vi "Dashboard Main.vi"() -> ()   [LabVIEW 2018]
uses:
  <vilib>/event_ctls.llb/eventvkey.ctl
  <vilib>/Rock Robotics/WPI/Dashboard/WPI_DashboardLogging Global.vi
  <vilib>/Utility/miscctls.llb/LVRowAndColumnTypeDef.ctl
  <vilib>/Rock Robotics/Network Tables/NT Read Boolean.vi
  7eadb382-1a2a-4737-94d3-f53f3babfc2e.vi
  <vilib>/Rock Robotics/Network Tables/NT Read Numeric Array.vi
  <vilib>/Utility/file.llb/Read Delimited Spreadsheet (string).vi
panel:
  in  "DB Camera Config 2":bool
  out "Camera Perf":string
  in  "Camera Settings":T1={"Frame Rate"=30, "Compression"=30, "Size"=1} {"Frame Rate" scale=1.0..30.0; "Compression" scale=100.0..-1.0; "Size" items=["640x480", "320x240", "160x120"]}
  in  "TCP":refnum<k5>
  out "Robot IP":string
  out "Image Message":string="Timeout in Camera Communications"
  in  "Dashboard Tab":T2(tab)
  in  "DB Camera Config":bool
  out "NT Connection":bool
  out "MotorChart R":cluster{"Numeric":dbl, "Numeric":dbl}(graph)
  out "MotorChart L":cluster{"Numeric":dbl, "Numeric":dbl}(graph)
  out "MotorSliders R":cluster{"MotorSlide1":dbl, "MotorSlide2":dbl} {"MotorSlide2" scale=-1.0..1.0 scale format="%#_2e"; "MotorSlide1" scale=-1.0..1.0 scale format="%#_2e"}
  out "MotorSliders L":cluster{"MotorSlide1":dbl, "MotorSlide2":dbl} {"MotorSlide2" scale=-1.0..1.0 scale format="%#_2e"; "MotorSlide1" scale=-1.0..1.0 scale format="%#_2e"}
  out "JS1 Z":dbl(slide) scale=-1.0..1.0 scale format="%#_2e"
  out "JS1 Graph":cluster{"X":dbl, "Y":dbl}[](graph)
  out "JS1 Buttons":T3
  out "JS2 Z":dbl(slide) scale=-1.0..1.0 scale format="%#_2e"
  out "JS2 Graph":cluster{"X":dbl, "Y":dbl}[](graph)
  out "JS2 Buttons":T3
  out "Mode":T4(ring)=enum."Auto Disabled"
  out "Right Camera Perf":cluster{"Bandwidth (Mbps)":dbl, "FPS":dbl}
  in  "Camera Name Right":string(combo)="No Camera Selection"
  in  "Camera Settings Right":T1={"Frame Rate"=30, "Compression"=30, "Size"=1} {"Frame Rate" scale=1.0..30.0; "Compression" scale=100.0..-1.0; "Size" items=["640x480", "320x240", "160x120"]}
  in  "Rec Mode":enum32{"Stop", "Record", "Playback"}(radio)
  in  "RIGHT TRAIN file path for Motion Profile Tester":path=path "C:/Users/Robotics/Desktop/2019 Deep Space/Motion Profile Examples and Resources/Phoenix-Examples-LabVIEW-master/MotionProfile (Edited by Drake)/mp.csv"
  out "RIGHT Trajectory Pts from .csv File":dbl[][](array[numeric])
  in  "Read New Profile for Tester":bool
  in  "LEFT TRAIN file path for Motion Profile Tester":path=path "C:/Users/Robotics/Desktop/2019 Deep Space/Motion Profile Examples and Resources/Phoenix-Examples-LabVIEW-master/MotionProfile (Edited by Drake)/mp.csv"
  out "LEFT Trajectory Pts from .csv File":dbl[][](array[numeric])
  out "Camera Image Right":T5(plugin-control)
  out "Front Limit \nSwitch":bool
  out "Back Limit\n Switch":bool
  in  "Select Auto":string(combo)="Select Autonomous ..."
  in  "DB/String 9":string
  in  "DB/String 8":string
  in  "DB/String 7":string
  in  "DB/String 6":string
  in  "DB/String 5":string
  in  "DB/String 4":string
  in  "DB/String 3":string
  in  "DB/String 2":string
  in  "DB/String 1":string
  in  "DB/String 0":string
  in  "DB/Slider 0":dbl(slide) scale=0.0..5.0
  in  "DB/Slider 1":dbl(slide) scale=0.0..5.0
  in  "DB/Slider 2":dbl(slide) scale=0.0..5.0
  in  "DB/Slider 3":dbl(slide) scale=0.0..5.0
  out "DB/LED 3":bool
  out "DB/LED 2":bool
  out "DB/LED 1":bool
  out "DB/LED 0":bool
  in  "DB/Button 3":bool
  in  "DB/Button 2":bool
  in  "DB/Button 1":bool
  in  "DB/Button 0":bool caption="New Name"
  in  "Test Slider":dbl(slide) scale=0.0..100.0 scale format="%#_3g"
  in  "On/Off":bool caption="Solenoid"
  in  "Test Name":u16(ring) items=["Select the test to run..."]
  in  "Test Tree":string(tree)
  in  "Motor":cluster{"Value":dbl, "Enable":bool} {"Value" scale=-1.0..1.0 scale format="%#_3g"}
  out "Progress":T6 {"Test Progress" scale=0.0..100.0}
  in  "Rev/Fwd":cluster{"Forward":bool, "Reverse":bool}
  in  "Test Ring":u16(ring) items=["Monochrome", "Color"]
  out "Cmd Status":string
  in  "Execute Command":bool
  in  "Command Params":string[][](table)
  in  "Command Selection":i32(listbox)
  in  "CheckList":i32(listbox)
  out "Tree":string(tree)
  out "Camera Image":T5(plugin-control)
  in  "Camera Name":string(combo)="No Camera Selection"
  # "HW"
  # "Joysticks"
  # "Drive Motors"
  # "Front"
  # "Right"
  # "Left"
  # "Back"
  # "HW"
  # "This tab is a great place for autonomous settings and robot-specific values.\nPlace controls and indicators inside this tab and match name to\nDashboard Variables on robot. You can also delete this comment."
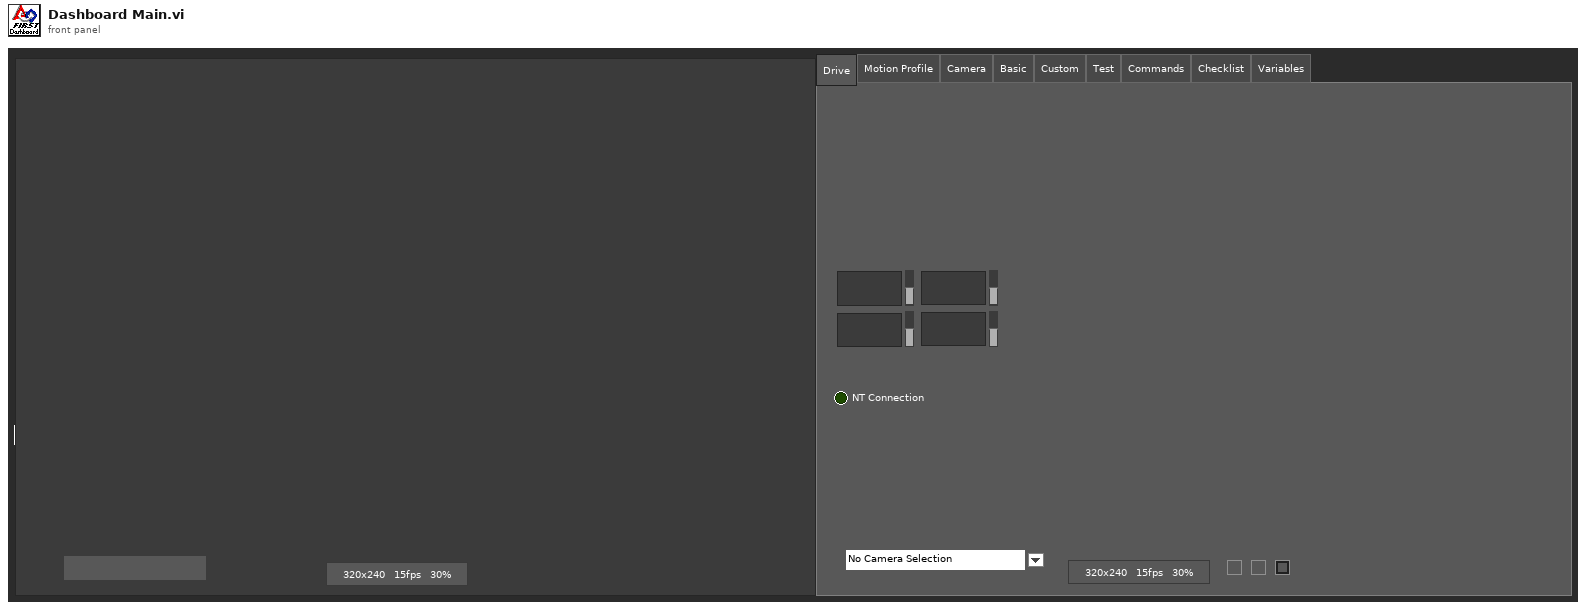
[diagram p1: front panel]
types:
  T1 = cluster{"Frame Rate":i32, "Compression":i32, "Size":u16}
  T2 = enum32{"Drive", "Motion Profile", "Camera", "Basic", "Custom", "Test", "Commands", "Checklist", "Variables"}
  T3 = cluster{bool, bool, bool, bool, bool, bool, bool, bool, bool, bool, bool, bool}
  T4 = enum8{"Tele-Op Disabled", "Tele-Op Enabled", "Auto Disabled", "Auto Enabled", "Test Disabled", "Test Enabled", "Disconnected", "No Code", "E-Stop"}
  T5 = typedef "IMAQ Image.ctl" = refnum<image>
  T6 = cluster{"Test Progress":u8, "Test Progress Text":string}
  T7 = cluster{"Save Path":path, "Interval (s)":dbl, "Keep":i32}
  T8 = enum32{"Drive", "Camera", "Basic", "Custom", "Test", "Commands", "Checklist", "Variables"}
  T9 = typedef "Image Type" = u32
  T10 = cluster{"IDs":cluster{"RPC field ID":u16, "Unique ID":u16}, "String":string}
  T11 = cluster{"Error Strings":string, "Disable Counts":cluster{u16, u16}, "Rail Faults":cluster{u16, u16, u16}, "Robot IP":string, "DB Mode":u8, "Event Info":cluster{"Name":string, "Type":u8, "Number":u16, "Replay":u8}}
  T12 = cluster{"Storage":cluster{"Disk Free":u64, "RAM Block":u32, "RAM free":u32}, "CPU Utilization":cluster{"CPU % ISR":sgl, "CPU % Time Crit":sgl, "CPU % Timed Str":sgl, "CPU % High":sgl, "CPU % Above":sgl, "CPU % Normal":sgl, "CPU % Low":sgl}, "CAN":cluster{"% Bus Utilization":sgl, "Bus Off Cnt":u32, "TX_FIFO Full Cnt":u32, "Receive Error Cnt":u8, "Transmit Error Cnt":u8}, "HID":cluster{"HID Outputs":u32, "Rumble Low":u16, "Rumble High":u16}[]}
  T13 = cluster{"Status bits":cluster{"Test Mode":bool, "Autonomous":bool, "Enabled":bool, "Code Start":bool, "Brownout":bool, "Reserved 2":bool, "Reserved 3":bool, "E-Stop":bool}, "Code Trace":cluster{"Disabled":bool, "TeleOp":bool, "Auto":bool, "Test":bool}, "Controller Type":enum16{"unknown", "cRIO", "roboRio"}, "Code?":enum16{"unknown", "noCode", "code"}, "Battery V":dbl}
  T14 = cluster{"Control Bits":cluster{"TestMode":bool, "Autonomous":bool, "Enabled":bool, "FMS Present":bool, bool, bool, bool, "E-Stop":bool}, "Team Station ":u8, "Countdown":sgl, "Joystick Values":cluster{"Axes":dbl[], "Buttons":bool[], "POVs":i16[]}[]}
  T15 = cluster{"Axes":dbl[], "Buttons":bool[], "POVs":i16[]}[]
  T16 = cluster{"Axes":dbl[], "Buttons":bool[], "POVs":i16[]}
  T17 = cluster{"Buttons[0]":bool, "Buttons[1]":bool, "Buttons[2]":bool, "Buttons[3]":bool, "Buttons[4]":bool, "Buttons[5]":bool, "Buttons[6]":bool, "Buttons[7]":bool, "Buttons[8]":bool, "Buttons[9]":bool, "Buttons[10]":bool, "Buttons[11]":bool}
  T18 = cluster{"Global Rectangle":i32[], "Contours":cluster{"Contour Type":u32, "ROI Type":u32, "Points":i32[]}[]}
  T19 = cluster{"Camera Name":string, string, "Saved DB Images Info":cluster{"Save Path":path, "Interval (s)":dbl, "Keep":i32}}
  T20 = cluster{"Camera Name Right":string, string, "Saved DB Images Info":cluster{"Save Path":path, "Interval (s)":dbl, "Keep":i32}}
  T21 = cluster{"Operation":enum16{"Update", "Clear"}, "Color Box":u32}[]
  T22 = typedef "eventvkey.ctl" = enum16{"ASCII", "Enter", "Return", "Shift", "Ctrl", "Alt", "Cmd", "Opt", "Caps", "NumLock", "Clear", "Break", "Up", "Down", "Left", "Right", "Insert", "Delete", "Home", "End", "PageUp", "PageDown", "Escape", "Help", "Pause", "ScrollLock", "F1", "F2", "F3", "F4", "F5", "F6", "F7", "F8", "F9", "F10", "F11", "F12", "F13", "F14", "F15", "F16", "F17", "F18", "F19", "F20", "F21", "F22", "F23", "F24", "Play", "VolumeUp", "VolumeDown", "Mute", "Two Byte Char"}
  T23 = cluster{"Image Size":bool, "Image Type":bool, "Pixel Value":bool, "ROI Information":bool, "Zoom Factor":bool}
  T24 = cluster{"Operation":enum16{"Update", "Clear"}, "Color Box":u32}
  T25 = typedef "LVRowAndColumnTypeDef.ctl" = cluster{"Row":i32, "Column":i32}
  T26 = cluster{"Shift":bool, "Ctrl":bool, "Alt":bool, "Cmd":bool, "Opt":bool}
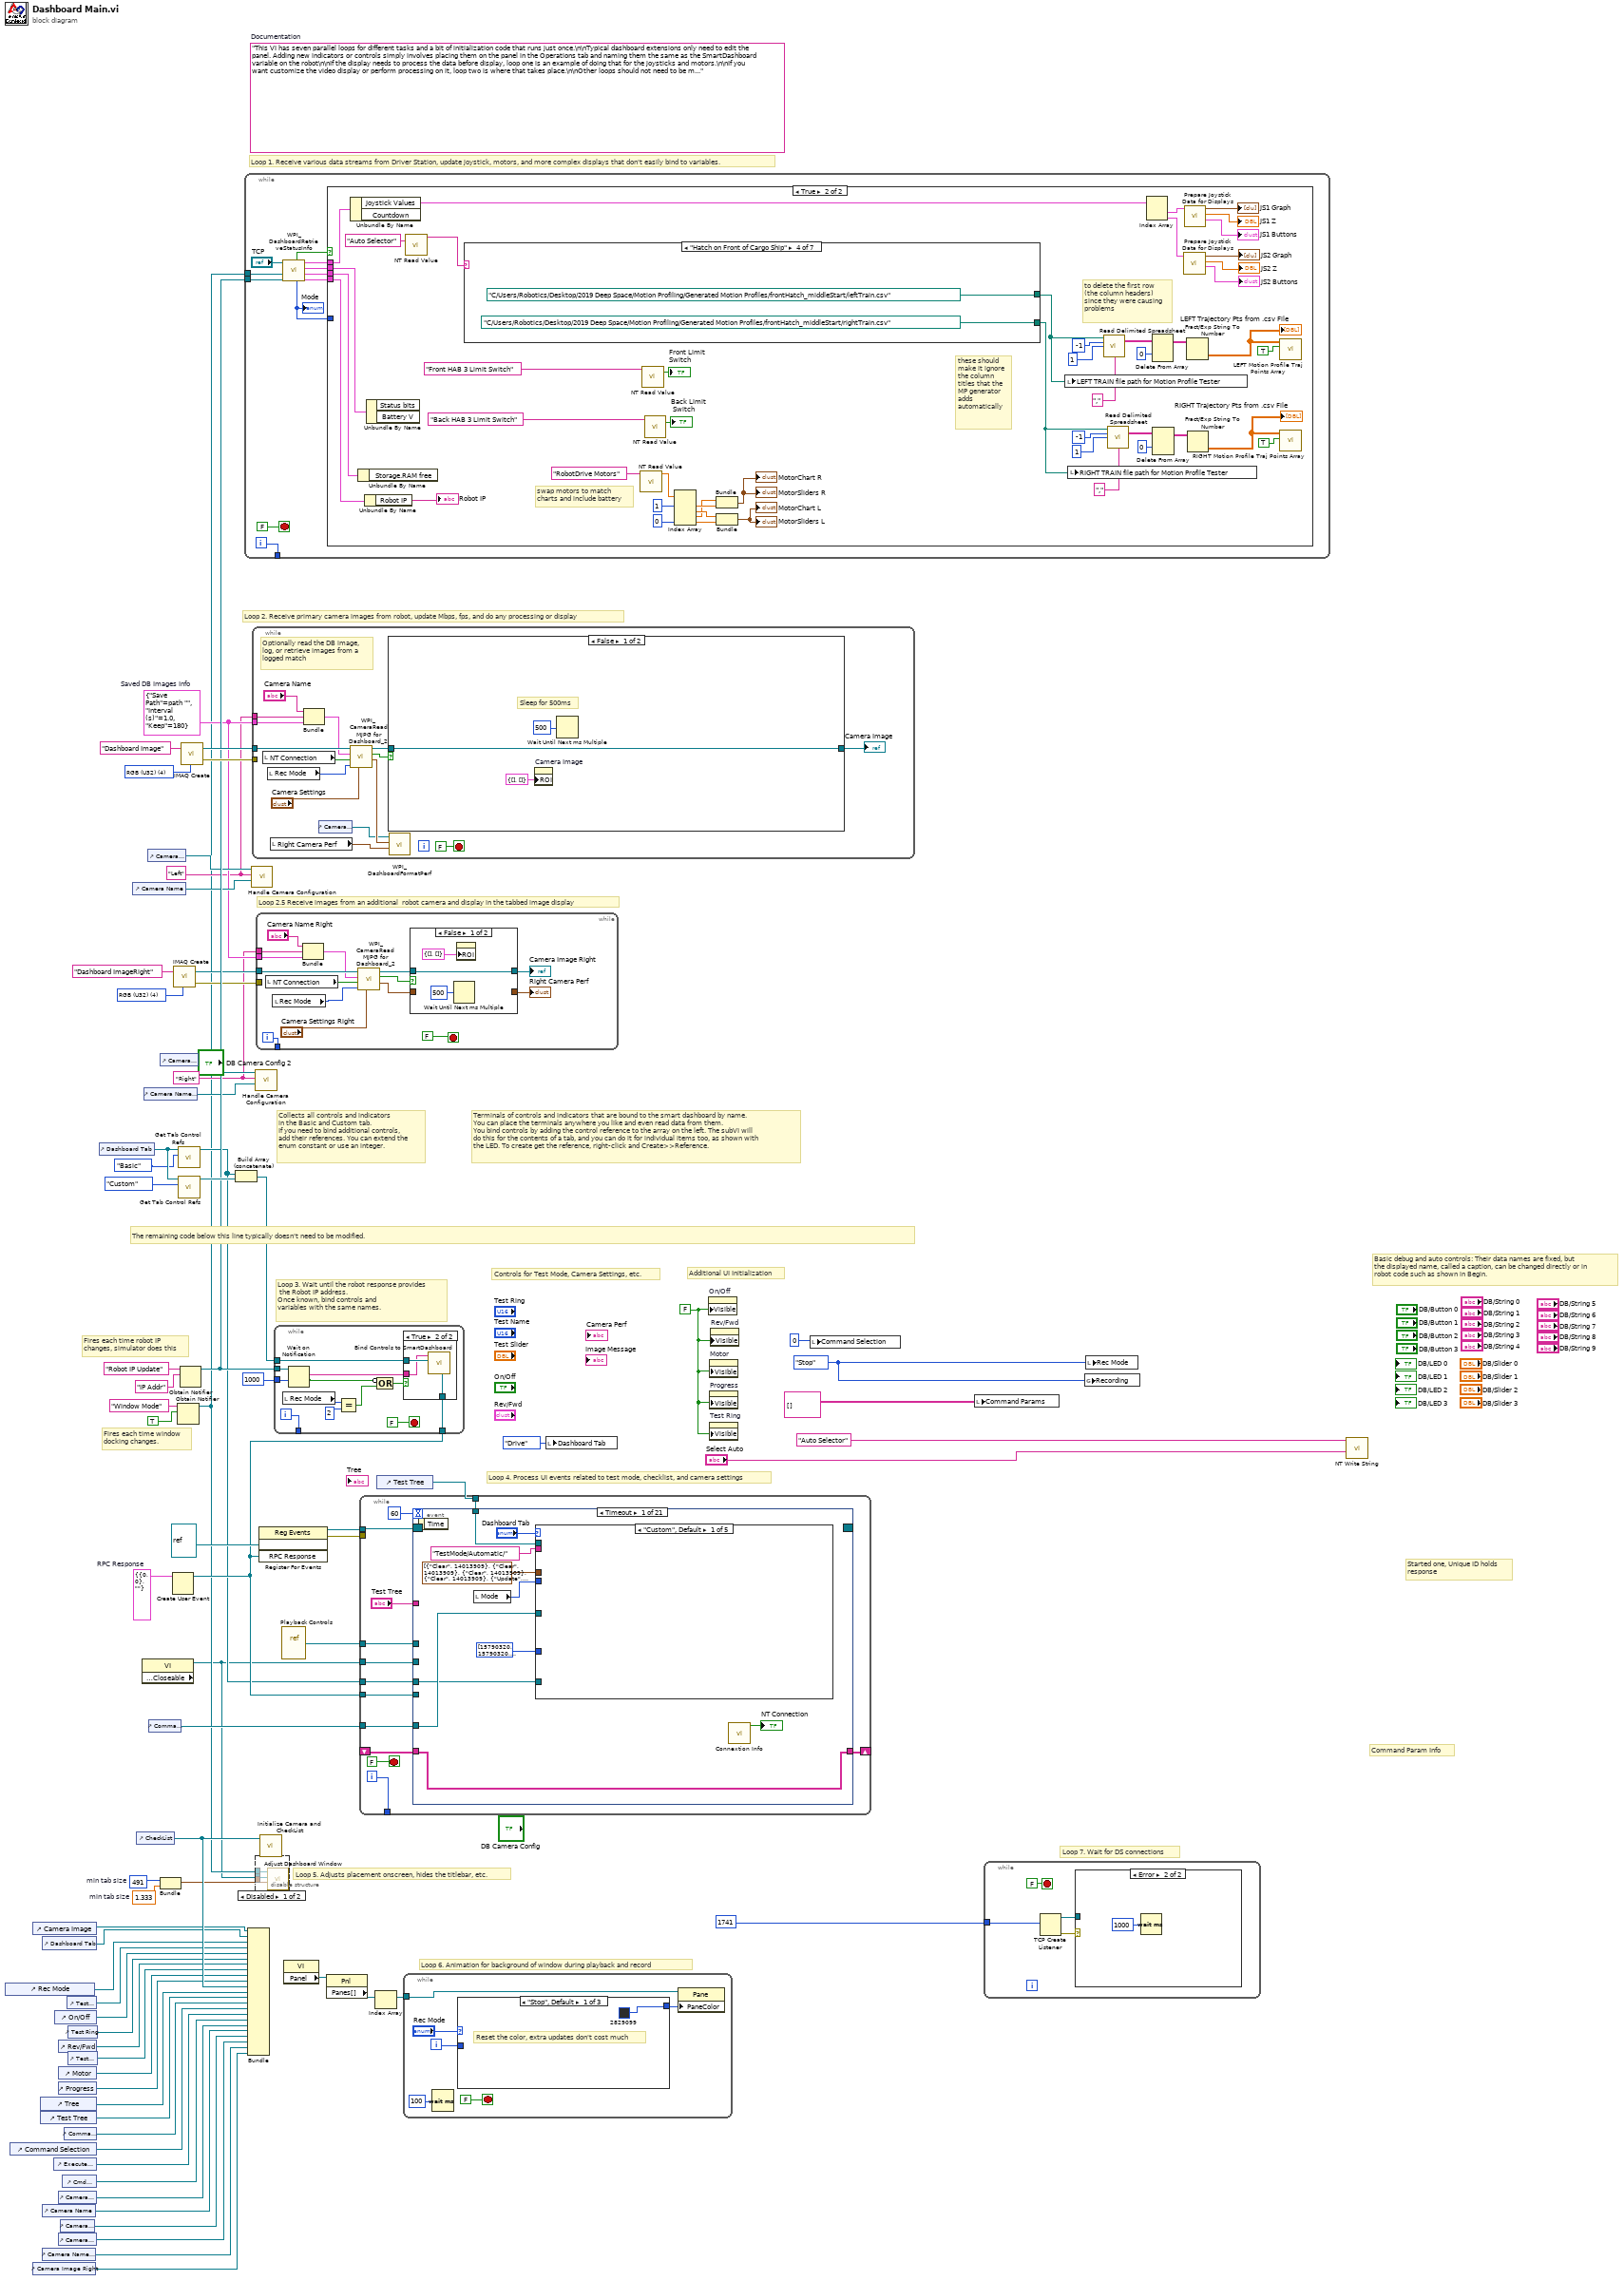
[diagram p0: block diagram]
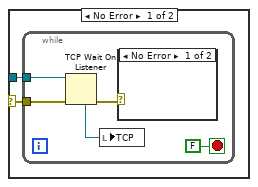
[diagram p4: hidden frame]
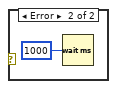
[diagram p5: hidden frame]
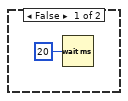
[diagram p6: hidden frame]
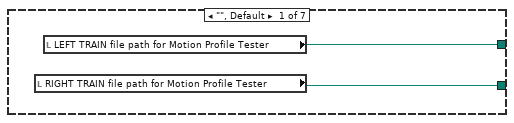
[diagram p7: hidden frame]
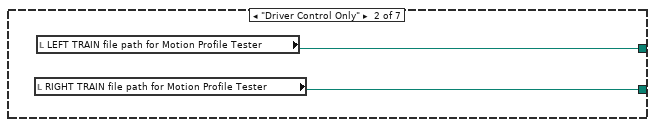
[diagram p8: hidden frame]
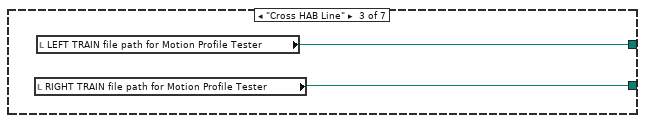
[diagram p9: hidden frame]
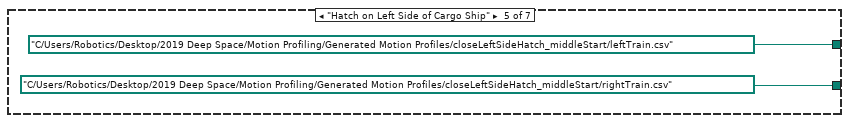
[diagram p10: hidden frame]
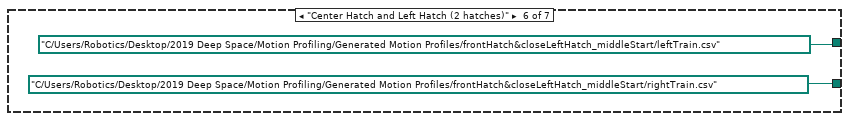
[diagram p11: hidden frame]
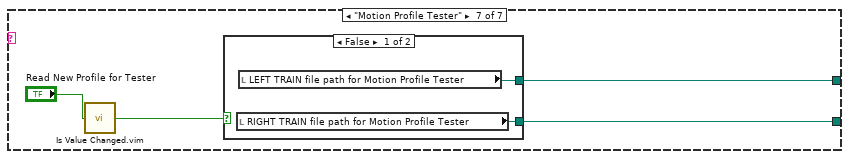
[diagram p12: hidden frame]
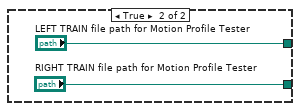
[diagram p13: hidden frame]
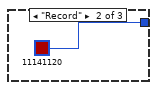
[diagram p14: hidden frame]
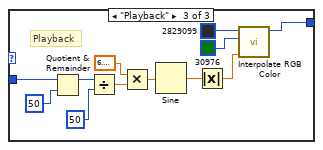
[diagram p15: hidden frame]
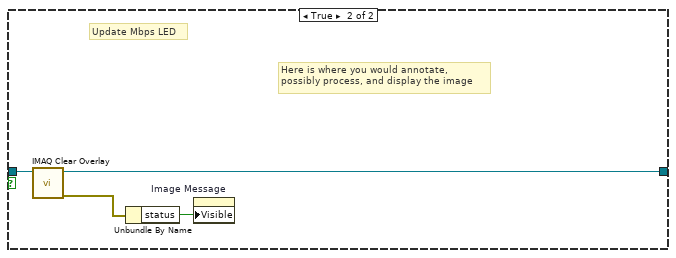
[diagram p17: hidden frame]
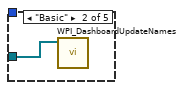
[diagram p18: hidden frame]
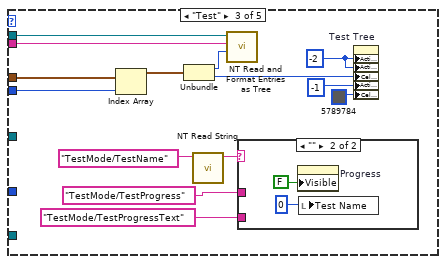
[diagram p19: hidden frame]
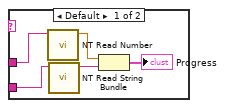
[diagram p20: hidden frame]
diagram:
  w9 = T7 {"Save Path"=path "", "Interval (s)"=1.0, "Keep"=180}  # Saved DB Images Info
  w8 = "Right"
  w7 = "Left"
  w19 = T9 4 items=["Grayscale (U8)", "Grayscale (I16)", "Grayscale (SGL)", "Complex (CSG)", "RGB (U32)", "HSL (U32)", "RGB (U64)"] ("Image Type")
  w35 = T10 {"IDs"={"RPC field ID"=0, "Unique ID"=0}, "String"=""}  # RPC Response
  w53 = 491  # min tab size
  w52 = 1.333  # min tab size
  w57 = enum32{"Stop", "Record", "Playback"}."Stop" ("Rec Mode")
  w40 = FALSE ("Visible")
  (unwired) "This VI has seven parallel loops for different tasks and a bit of initialization code that runs just once.\n\nTypical dashboard extensions only need to edit the panel. Adding new indicators or controls simply involves placing them on the panel in the Operations tab and naming them the same as the SmartDashboard variable on the robot\n\nIf the display needs to process the data before display, loop one is an example of doing that for the joysticks and motors.\n\nIf you want customize the video display or perform processing on it, loop two is where that takes place.\n\nOther loops should not need to be modified. They are pretty standard, and document the task they perform."  # Documentation
  w74 = T9 4 items=["Grayscale (U8)", "Grayscale (I16)", "Grayscale (SGL)", "Complex (CSG)", "RGB (U32)", "HSL (U32)", "RGB (U64)"] ("Image Type")
  # "Loop 5. Adjusts placement onscreen, hides the titlebar, etc."
  # "Loop 2.5 Receive images from an additional  robot camera and display in the tabbed image display"
  # "Command Param Info"
  # "Started one, Unique ID holds\nresponse"
  # "Loop 7. Wait for DS connections"
  # "Basic debug and auto controls: Their data names are fixed, but\nthe displayed name, called a caption, can be changed directly or in\nrobot code such as shown in Begin."
  # "Controls for Test Mode, Camera Settings, etc."
  # "Additional UI Initialization"
  # "Loop 6. Animation for background of window during playback and record"
  # "Fires each time robot IP\nchanges, simulator does this"
  # "Fires each time window\ndocking changes."
  # "Collects all controls and indicators\nin the Basic and Custom tab.\nIf you need to bind additional controls,\nadd their references. You can extend the\nenum constant or use an integer."
  # "The remaining code below this line typically doesn't need to be modified."
  # "Loop 4. Process UI events related to test mode, checklist, and camera settings"
  # "Terminals of controls and indicators that are bound to the smart dashboard by name.\nYou can place the terminals anywhere you like and even read data from them.\nYou bind controls by adding the control reference to the array on the left. The subVI will\ndo this for the contents of a tab, and you can do it for individual items too, as shown with\nthe LED. To create get the reference, right-click and Create>>Reference."
  # "Loop 3. Wait until the robot response provides\n the Robot IP address.\nOnce known, bind controls and\nvariables with the same names."
  # "Loop 1. Receive various data streams from Driver Station, update joystick, motors, and more complex displays that don't easily bind to variables."
  # "Loop 2. Receive primary camera images from robot, update Mbps, fps, and do any processing or display"
  n1 = control-ref of="Rec Mode"() -> (w46:refnum<vi>)
  n2 = control-ref of="Command Selection"() -> (w34:refnum<vi>)
  n3 = control-ref of="Camera Image Right"() -> (w12:refnum<vi>)
  n4 = control-ref of="Camera Image"() -> (w5:refnum<vi>)
  n5 = control-ref of="Tree"() -> (w50:refnum<vi>)
  n6 = control-ref of="Test Tree"() -> (w49:refnum<vi>)
  n7 = control-ref of="Dashboard Tab"() -> (w6:refnum<vi>)
  n8 = control-ref of="Camera Name"() -> (w25:refnum<vi>)
  n9 = control-ref of="Camera Name Right"() -> (w13:refnum<vi>)
  n10 = control-ref of="Execute Command"() -> (w36:refnum<vi>)
  n11 = control-ref of="On/Off"() -> (w44:refnum<vi>)
  n12 = control-ref of="Progress"() -> (w41:refnum<vi>)
  n13 = control-ref of="Camera Settings"() -> (w26:refnum<vi>)
  n14 = control-ref of="Camera Settings Right"() -> (w14:refnum<vi>)
  n15 = control-ref of="Rev/Fwd"() -> (w42:refnum<vi>)
  n16 = control-ref of="Motor"() -> (w47:refnum<vi>)
  n17 = control-ref of="Camera Perf"() -> (w24:refnum<vi>)
  n18 = control-ref of="Cmd Status"() -> (w30:refnum<vi>)
  n19 = control-ref of="Command Params"() -> (w37:refnum<vi>)
  n20 = control-ref of="Test Slider"() -> (w45:refnum<vi>)
  n21 = control-ref of="Test Ring"() -> (w43:refnum<vi>)
  n22 = control-ref of="Test Name"() -> (w48:refnum<vi>)
  n23 = control-ref of="Dashboard Tab"() -> (w56:refnum<vi>)
  n24 = control-ref of="Camera Name"() -> (w27:refnum<vi>)
  n25 = control-ref of="CheckList"() -> (w51:refnum<vi>)
  n26 = property class="VI" props=["Front Panel.Closeable"]() -> (reference out=w2:refnum<vi>)  [unwired: 2 in, 2 out]
  n27 = control-ref of="Camera Name Right"() -> (w15:refnum<vi>)
  n28 = control-ref of="Camera Settings"() -> (w28:refnum<vi>)
  n29 = control-ref of="Command Params"() -> (w29:refnum<vi>)
  n30 = control-ref of="Camera Settings Right"() -> (w16:refnum<vi>)
  n31 = Bundle("min tab size"=w53, "min tab size"=w52) -> (w1:cluster{"min tab size":i32, "min tab size":dbl})  [unwired: 1 in]
  n32 = Create User Event(user event datatype=w35) -> (user event=w31:refnum<user-event>)  [unwired: 1 in, 1 out]
  n33 = call "IMAQ Create"("Image Name"="Dashboard ImageRight", "Image Type"=w19) -> ("New Image"=w18:T5, "error out"=w17:errorcluster)  [unwired: 2 in, 1 out]
  n34 = Obtain Notifier(name (unnamed)="Window Mode", notification data type=TRUE) -> (notifier out=w3:refnum<notifier>)  [unwired: 2 in, 2 out]
  n35 = call <vilib>:"Get Tab Control Refs.vi"("Page Index"=T8."Basic" ("Dashboard Tab"), "TabControl in"=w56) -> ("ControlsOnPage"=w23:refnum<vi>[])  [unwired: 9 in]
  n36 = call <vilib>:"Get Tab Control Refs.vi"("Page Index"=T8."Custom" ("Dashboard Tab"), "TabControl in"=w56) -> ("ControlsOnPage"=w55:refnum<vi>[])  [unwired: 9 in]
  n37 = Obtain Notifier(name (unnamed)="Robot IP Update", notification data type="IP Addr" ("name (unnamed)")) -> (notifier out=w39:refnum<notifier>)  [unwired: 2 in, 2 out]
  n38 = call "IMAQ Create"("Image Name"="Dashboard Image", "Image Type"=w74) -> ("New Image"=w72:T5, "error out"=w71:errorcluster)  [unwired: 2 in, 1 out]
  n39 = Build Array (concatenate)(w23, w55) -> (w54:refnum<vi>[])
  n40 = while {
    tunnel: [w84] -> _
    tunnel: w39 -> [w78]
    tunnel: w3 -> [w75]
    i -> [w84]
    stop <- FALSE stop-if-true
    n41 = call <vilib>:"WPI_DashboardRetrieveStatusInfo.vi"("Binding Refnum"=w78, "Window Mode Notifier"=w75, "TCP Cnx"="TCP") -> ("Power and Errors"=w79:T11, "Robot Metrics"=w82:T12, "Status Info"=w83:T13, "Control Info"=w80:T14, "Robot Mode"=w77:T4, "Process?"=w81:bool)  [unwired: 3 in]
    "Mode" <- w77
    n42 = case shown="True" w81 {
      tunnel: w83 -> [_ w134]
      tunnel: w82 -> [_ w133]
      tunnel: w80 -> [_ w132]
      tunnel: w79 -> [_ w131]
      tunnel: w77 -> [_ _]
      frame False {
        n43 = Wait (ms)(milliseconds to wait=u32 20) -> ()  [unwired: 1 out]
      }
      frame True {
        # "to delete the first row\n(the column headers) \nsince they were causing\nproblems"
        # "these should\nmake it ignore\nthe column \ntitles that the \nMP generator\nadds \nautomatically"
        # "swap motors to match\ncharts and include battery"
        n44 = Unbundle By Name(w132) -> ("Joystick Values"=w122:T15)  [unwired: 1 out]
        n45 = Unbundle By Name(w133) -> ()  [unwired: 1 out]
        n46 = Unbundle By Name(w131) -> ("Robot IP"=→"Robot IP":string)
        n47 = Unbundle By Name(w134) -> ()  [unwired: 2 out]
        n48 = call-poly <vilib>:"NT Read Value.vi"("Name"="Auto Selector") -> ("String"=w107:string)  [unwired: 9 in, 1 out]
        n49 = case shown="\"Hatch on Front of Cargo Ship\"" w107 {
          tunnel: [w136 w138 w139 path "C:/Users/Robotics/Desktop/2019 Deep Space/Motion Profiling/Generated Motion Profiles/frontHatch_middleStart/leftTrain.csv" path "C:/Users/Robotics/Desktop/2019 Deep Space/Motion Profiling/Generated Motion Profiles/closeLeftSideHatch_middleStart/leftTrain.csv" path "C:/Users/Robotics/Desktop/2019 Deep Space/Motion Profiling/Generated Motion Profiles/frontHatch&closeLeftHatch_middleStart/leftTrain.csv" w150] -> w97
          tunnel: [w135 w137 w140 path "C:/Users/Robotics/Desktop/2019 Deep Space/Motion Profiling/Generated Motion Profiles/frontHatch_middleStart/rightTrain.csv" path "C:/Users/Robotics/Desktop/2019 Deep Space/Motion Profiling/Generated Motion Profiles/closeLeftSideHatch_middleStart/rightTrain.csv" path "C:/Users/Robotics/Desktop/2019 Deep Space/Motion Profiling/Generated Motion Profiles/frontHatch&closeLeftHatch_middleStart/rightTrain.csv" w149] -> w103
          frame "", Default {
            n50 = local read "RIGHT TRAIN file path for Motion Profile Tester"() -> (w135:path)
            n51 = local read "LEFT TRAIN file path for Motion Profile Tester"() -> (w136:path)
          }
          frame "Driver Control Only" {
            n52 = local read "RIGHT TRAIN file path for Motion Profile Tester"() -> (w137:path)
            n53 = local read "LEFT TRAIN file path for Motion Profile Tester"() -> (w138:path)
          }
          frame "Cross HAB Line" {
            n54 = local read "RIGHT TRAIN file path for Motion Profile Tester"() -> (w140:path)
            n55 = local read "LEFT TRAIN file path for Motion Profile Tester"() -> (w139:path)
          }
          frame "Hatch on Front of Cargo Ship" {
          }
          frame "Hatch on Left Side of Cargo Ship" {
          }
          frame "Center Hatch and Left Hatch (2 hatches)" {
          }
          frame "Motion Profile Tester" {
            n56 = call "Is Value Changed.vim"("value"="Read New Profile for Tester") -> ("changed or first call?"=w147:bool)
            n57 = case shown="False" w147 {
              tunnel: [w152 "LEFT TRAIN file path for Motion Profile Tester"] -> w150
              tunnel: [w151 "RIGHT TRAIN file path for Motion Profile Tester"] -> w149
              frame False {
                n58 = local read "RIGHT TRAIN file path for Motion Profile Tester"() -> (w151:path)
                n59 = local read "LEFT TRAIN file path for Motion Profile Tester"() -> (w152:path)
              }
              frame True {
              }
            }
          }
        }
        n60 = call-poly <vilib>:"NT Read Value.vi"("Name"="RobotDrive Motors") -> ("Numeric Array"=w112:dbl[])  [unwired: 9 in, 1 out]
        n61 = call-poly <vilib>:"NT Read Value.vi"("Name"="Front HAB 3 Limit Switch") -> ("Boolean"=→"Front Limit \nSwitch":bool)  [unwired: 9 in, 1 out]
        n62 = call-poly <vilib>:"NT Read Value.vi"("Name"="Back HAB 3 Limit Switch") -> ("Boolean"=→"Back Limit\n Switch":bool)  [unwired: 9 in, 1 out]
        n63 = Index Array(array=w112, index #1=1, index #4=0) -> (element #1=w126:dbl, element #2=w127:dbl, element #3=w125:dbl, element #4=w130:dbl)  [unwired: 2 in]
        n64 = Bundle("Numeric"=w125, "Numeric"=w126) -> (→"MotorChart R" →"MotorSliders R":cluster{"Numeric":dbl, "Numeric":dbl})  [unwired: 1 in]
        n65 = Bundle("Numeric"=w127, "Numeric"=w130) -> (→"MotorChart L" →"MotorSliders L":cluster{"Numeric":dbl, "Numeric":dbl})  [unwired: 1 in]
        n66 = local write "LEFT TRAIN file path for Motion Profile Tester"(w97) -> ()
        n67 = local write "RIGHT TRAIN file path for Motion Profile Tester"(w103) -> ()
        n68 = call-poly <vilib>:"Read Delimited Spreadsheet.vi"("file path (dialog if empty)"=w97, "number of rows (all:-1)"=-1, "start of read offset (chars.:0)"=1, "delimiter (\\t)"="," ("delimiter (\\t)")) -> ("all rows"=w95:string[][])  [unwired: 6 in, 5 out]
        n69 = call-poly <vilib>:"Read Delimited Spreadsheet.vi"("file path (dialog if empty)"=w103, "number of rows (all:-1)"=-1, "start of read offset (chars.:0)"=1, "delimiter (\\t)"="," ("delimiter (\\t)")) -> ("all rows"=w90:string[][])  [unwired: 6 in, 5 out]
        n70 = Index Array(array=w122) -> (element #1=w121:T16, element #2=w117:T16)  [unwired: 2 in]
        n71 = Delete From Array(array=w95, index (row)=0 ("index")) -> (array with subset deleted=w94:string[][])  [unwired: 2 in, 1 out]
        n72 = Delete From Array(array=w90, index (row)=0 ("index")) -> (array with subset deleted=w91:string[][])  [unwired: 2 in, 1 out]
        n73 = call "Prepare Joystick Data for Displays.vi"("Joystick Values"=w117) -> ("Buttons"=→"JS2 Buttons":T17, "Z Axis"=→"JS2 Z":dbl, "Cartesian Data"=→"JS2 Graph":cluster{"X axis":dbl, "X axis":dbl}[])  [unwired: 8 in]
        n74 = call "Prepare Joystick Data for Displays.vi"("Joystick Values"=w121) -> ("Buttons"=→"JS1 Buttons":T17, "Z Axis"=→"JS1 Z":dbl, "Cartesian Data"=→"JS1 Graph":cluster{"X axis":dbl, "X axis":dbl}[])  [unwired: 8 in]
        n75 = Fract/Exp String To Number(string=w94) -> (number=w93:dbl[][])  [unwired: 3 in, 1 out]
        "LEFT Trajectory Pts from .csv File" <- w93
        n76 = Fract/Exp String To Number(string=w91) -> (number=w89:dbl[][])  [unwired: 3 in, 1 out]
        "RIGHT Trajectory Pts from .csv File" <- w89
        n77 = call "LEFT Motion Profile Traj Points Array.vi"("Read = false, Write = true"=TRUE, "traj. points array in"=w93) -> ()  [unwired: 9 in, 1 out]
        n78 = call "RIGHT Motion Profile Traj Points Array.vi"("Read = false, Write = true"=TRUE, "traj. points array in"=w89) -> ()  [unwired: 9 in, 1 out]
      }
    }
  }
  n79 = Bundle("Camera Image"=w5, "Dashboard Tab"=w6, "Rec Mode"=w46, "Test Slider"=w45, "On/Off"=w44, "Test Ring"=w43, "Rev/Fwd"=w42, "Test Name"=w48, "Motor"=w47, "Progress"=w41, "CheckList"=w51, "Tree"=w50, "Test Tree"=w49, "Command Params"=w37, "Command Selection"=w34, "Execute Command"=w36, "Cmd Status"=w30, "Camera Settings"=w26, "Camera Name"=w25, "Camera Perf"=w24, "Camera Settings Right"=w14, "Camera Name Right"=w13, "Camera Image Right"=w12) -> ()  [unwired: 1 in, 1 out]
  n80 = call "Handle Camera Configuration.vi"("CameraNameRef"=w27, "Display Name"=w7, "ClusterRef"=w28) -> ()  [unwired: 9 in]
  n81 = while {
    tunnel: w72 -> [w168]
    tunnel: w71 -> [_]
    tunnel: w9 -> [w161]
    tunnel: w7 -> [w158]
    stop <- FALSE stop-if-true
    # "Optionally read the DB image,\nlog, or retrieve images from a\nlogged match"
    n82 = local read "NT Connection"() -> (w162:bool)
    n83 = local read "Rec Mode"() -> (w165:enum32{"Stop", "Record", "Playback"})
    n84 = local read "Right Camera Perf"() -> (w156:cluster{"Bandwidth (Mbps)":dbl, "FPS":dbl})
    n85 = Bundle("Camera Name"="Camera Name", w158, "Saved DB Images Info"=w161) -> (w160:T19)  [unwired: 1 in]
    n86 = control-ref of="Camera Perf"() -> (w155:refnum<vi>)
    n87 = call <vilib>:"WPI_CameraRead MJPG for Dashboard_2.vi"("Camera Settings"="Camera Settings", "Rec Mode"=w165, "NT Connection"=w162, "Capture Info"=w160, "Image in"=w168) -> ("perf info"=w157:cluster{"Bandwidth (Mbps)":dbl, "fps":dbl}, "Active"=w166:bool, "Image\\ out"=w167:T5)  [unwired: 4 in]
    n88 = case shown="False" w166 {
      tunnel: w167 -> [w171 w174]
      tunnel: [w171 w173] -> w163
      frame False {
        # "Sleep for 500ms"
        n89 = property on="Camera Image" class="ImageControl"("ROI"=T18 {"Global Rectangle"=[], "Contours"=[]}) -> ()  [unwired: 2 in, 2 out]
        n90 = Wait Until Next ms Multiple(millisecond multiple=u32 500) -> ()  [unwired: 1 out]
      }
      frame True {
        # "Here is where you would annotate,\npossibly process, and display the image"
        # "Update Mbps LED"
        n91 = call "IMAQ Clear Overlay"("Image"=w174) -> ("error out"=w175:errorcluster, "Image Out"=w173:T5)  [unwired: 2 in, 7 out]
        n92 = Unbundle By Name(w175) -> ("status"=w176:bool)
        n93 = property on="Image Message" class="Str"("Visible"=w176) -> ()  [unwired: 2 in, 2 out]
      }
    }
    "Camera Image" <- w163
    n94 = call <vilib>:"WPI_DashboardFormatPerf.vi"("Right Camera Perf"=w156, "Performance"=w157, "String in"=w155) -> ()  [unwired: 9 in]
  }
  n95 = disable-structure shown="Disabled" {
    disable-tunnel: w3 -> [w179 _]
    disable-tunnel: w2 -> [w178 _]
    disable-tunnel: w1 -> [w177 _]
    frame Disabled {
      n96 = call "Adjust Dashboard Window.vi"("Size Constraints"=w177, "VI"=w178, "WIn Mode"=w179) -> ()  [unwired: 9 in]
    }
    frame Enabled {
    }
  }
  n97 = call "Handle Camera Configuration.vi"("CameraNameRef"=w15, "Display Name"=w8, "ClusterRef"=w16) -> ()  [unwired: 9 in]
  n98 = while {
    tunnel: w18 -> [w194]
    tunnel: w17 -> [_]
    tunnel: [w189] -> _
    tunnel: w9 -> [w185]
    tunnel: w8 -> [w182]
    i -> [w189]
    stop <- FALSE stop-if-true
    n99 = local read "NT Connection"() -> (w186:bool)
    n100 = local read "Rec Mode"() -> (w193:enum32{"Stop", "Record", "Playback"})
    n101 = Bundle("Camera Name Right"="Camera Name Right", w182, "Saved DB Images Info"=w185) -> (w184:T20)  [unwired: 1 in]
    n102 = call <vilib>:"WPI_CameraRead MJPG for Dashboard_2.vi"("Camera Settings"="Camera Settings Right", "Rec Mode"=w193, "NT Connection"=w186, "Capture Info"=w184, "Image in"=w194) -> ("perf info"=w180:cluster{"Bandwidth (Mbps)":dbl, "fps":dbl}, "Active"=w188:bool, "Image\\ out"=w191:T5)  [unwired: 4 in]
    n103 = case shown="False" w188 {
      tunnel: w191 -> [w196 w199]
      tunnel: [w196 w199] -> w187
      tunnel: [_ w198] -> w181
      tunnel: w180 -> [_ w198]
      frame False {
        n104 = Wait Until Next ms Multiple(millisecond multiple=u32 500) -> ()  [unwired: 1 out]
        n105 = property on="Camera Image Right" class="ImageControl"("ROI"=T18 {"Global Rectangle"=[], "Contours"=[]}) -> ()  [unwired: 2 in, 2 out]
      }
      frame True {
      }
    }
    "Camera Image Right" <- w187
    "Right Camera Perf" <- w181
  }
  n106 = register-events(refnum<vi> refnum, w31) -> (reference out=w61:refnum<event-registration>, error out=w60:errorcluster)  [unwired: 2 in]
  n107 = call "Initialize Camera and CheckList.vi"("ListBox in"=w51) -> ()  [unwired: 11 in]
  n108 = while {
    tunnel: w54 -> [w211]
    tunnel: w39 -> [w209]
    tunnel: [w207] -> _
    tunnel: u32 1000 ("milliseconds to wait") -> [w206]
    tunnel: w31 -> [w200]
    i -> [w207]
    stop <- FALSE stop-if-true
    n109 = local read "Rec Mode"() -> (w202:enum32{"Stop", "Record", "Playback"})
    n110 = Wait on Notification(notifier=w209, timeout in ms (-1)=w206) -> (notification=w208:string, timed out?=w204:bool)  [unwired: 2 in, 2 out]
    n111 = Equal?(x=w202, y=u16 2 ("Rec Mode")) -> (x = y?=w203:bool)
    n112 = Compound Arithmetic op=OR(invert w204, w203) -> (w205:bool)
    n113 = case shown="True" w205 {
      tunnel: w211 -> [_ w214]
      tunnel: w208 -> [_ w213]
      tunnel: w200 -> [_ w212]
      frame False {
      }
      frame True {
        n114 = call <vilib>:"Bind Controls to SmartDashboard.vi"("RPC ref"=w212, "Bound Control Refs"=w214, "Server IP Address"=w213) -> ()  [unwired: 9 in]
      }
    }
  }
  n115 = vi-ref "Playback Controls.vi"() -> (w62:refnum<vi>)
  n116 = property class="VI"() -> ("Panel"=w64:refnum<vi>)  [unwired: 2 in, 2 out]
  n117 = property class="Pnl"(reference=w64) -> ("Panes[]"=w65:refnum<vi>[])  [unwired: 1 in, 2 out]
  n118 = Index Array(array=w65) -> (element=w63:refnum<vi>)  [unwired: 1 in]
  n119 = control-ref of="Test Tree"() -> (w66:refnum<vi>)
  n120 = while {
    tunnel: [w224] -> _
    tunnel: w66 -> [w223]
    tunnel: w62 -> [w222]
    tunnel: w61 -> [w221]
    tunnel: w60 -> [_]
    tunnel: w2 -> [w220]
    tunnel: w31 -> [w219]
    tunnel: w29 -> [w218]
    shift-right: [w217] -> _
    shift-left: _ -> [w216]
    tunnel: w23 -> [w215]
    i -> [w224]
    stop <- FALSE stop-if-true
    n121 = event shown="[0] Timeout" {
      selector: w221 -> [_ _ _ _ _ _ _ _ _ _ _ _ _ _ _ _ _ _ _ _ _]
      dyn-events: [_ _ _ _ _ _ _ _ _ _ _ _ _ _ _ _ w484 _ _ _ _] -> _
      timeout: u32 60 ("milliseconds to wait") -> [_ _ _ _ _ _ _ _ _ _ _ _ _ _ _ _ _ _ _ _ _]
      tunnel: w223 -> [w236 _ _ _ _ _ _ _ _ _ _ _ _ _ _ _ _ _ _ _ _]
      tunnel: "Test Tree" -> [_ _ _ _ _ _ _ _ _ _ _ w451 w459 w461 w465 w473 _ _ _ _ _]
      tunnel: w222 -> [_ _ _ _ _ _ _ _ _ _ _ _ _ _ _ _ w486 _ w504 _ _]
      tunnel: w220 -> [_ _ _ _ _ _ _ _ _ _ _ _ _ _ _ _ w482 _ _ _ _]
      tunnel: w219 -> [_ _ _ _ _ _ _ _ _ _ _ _ _ _ _ _ w480 _ _ _ _]
      tunnel: w218 -> [w231 _ _ _ _ _ w402 _ _ _ _ _ _ _ _ _ _ _ _ _ _]
      tunnel: [w230 w279 w381 w386 w395 w399 w400 w409 w419 w426 w438 w450 w457 w460 w464 w472 w479 w499 w501 w505 w518] -> w217
      tunnel: w216 -> [w230 w279 w381 w386 w395 w399 w400 _ _ w426 w438 w450 w457 w460 w464 w472 w479 w499 w501 w505 w518]
      tunnel: w215 -> [w228 _ _ _ _ _ _ _ _ _ _ _ _ _ _ _ _ _ _ _ _]
      event Timeout {
        n122 = event-data() -> ()  [unwired: 1 in, 1 out]
        n123 = local read "Mode"() -> (w233:T4)
        n124 = case shown="\"Custom\", Default" "Dashboard Tab" {
          tunnel: w236 -> [_ _ w252 _ _]
          tunnel: "TestMode/Automatic/" ("Name Pattern") -> [_ _ w251 _ _]
          tunnel: T21 [{"Operation"=enum."Clear", "Color Box"=14013909}, {"Operation"=enum."Clear", "Color Box"=14013909}, {"Operation"=enum."Clear", "Color Box"=14013909}, {"Operation"=enum."Clear", "Color Box"=14013909}, {"Operation"=enum."Update", "Color Box"=14013909}, {"Operation"=enum."Update", "Color Box"=16777215}, {"Operation"=enum."Clear", "Color Box"=14013909}, {"Operation"=enum."Clear", "Color Box"=14013909}, {"Operation"=enum."Clear", "Color Box"=14013909}] -> [_ _ w244 _ w272]
          tunnel: w233 -> [_ _ w243 _ w271]
          tunnel: u32[] [15790320, 15790320, 15790320, 15790320, 16777215, 16777215, 15790320, 15790320, 15790320] -> [_ _ _ _ w277]
          tunnel: w231 -> [_ _ _ _ w265]
          tunnel: w228 -> [_ w238 _ _ _]
          frame "Custom", Default {
          }
          frame "Basic" {
            n125 = call <vilib>:"WPI_DashboardUpdateNames.vi"("Controls on Tab"=w238) -> ()  [unwired: 11 in]
          }
          frame "Test" {
            w250 = -2 ("Active Item:Row Number")
            n126 = Index Array(array=w244, index=w243) -> (element=w245:T24)
            n127 = Unbundle(w245) -> ("Operation"=w246:enum16{"Update", "Clear"}, "Color Box"=w247:u32)
            n128 = call <vilib>:"NT Read String.vi"("Name"="TestMode/TestName") -> ("String"=w241:string)  [unwired: 9 in, 1 out]
            n129 = call <vilib>:"NT Read and Format Entries as Tree.vi"("Operation"=w246, "Name Pattern"=w251, "Tree Refnum"=w252) -> ()  [unwired: 7 in, 2 out]
            n130 = case shown="\"\"" w241 {
              tunnel: "TestMode/TestProgress" ("Name") -> [w254 _]
              tunnel: "TestMode/TestProgressText" ("Name") -> [w253 _]
              frame Default {
                n131 = call <vilib>:"NT Read Number.vi"("Name"=w254) -> ("Numeric"=w255:dbl)  [unwired: 9 in, 1 out]
                n132 = call <vilib>:"NT Read String.vi"("Name"=w253) -> ("String"=w256:string)  [unwired: 9 in, 1 out]
                n133 = Bundle("Numeric"=w255, "String"=w256) -> (→"Progress":cluster{"Numeric":dbl, "String":string})  [unwired: 1 in]
              }
              frame "" {
                n134 = property on="Progress" class="Clust (strict)"("Visible"=FALSE) -> ()  [unwired: 2 in, 2 out]
                n135 = local write "Test Name"(u16 0) -> ()
              }
            }
            n136 = property on="Test Tree" class="Tree (strict)"("Active Item Row Number"=w250, "ActiveColNum"=w250, "CellBG"=w247, "Active Item Row Number"=-1 ("Active Item:Row Number"), "CellBG"=u32 5789784 ("Color Box")) -> ()  [unwired: 2 in, 2 out]
          }
          frame "Variables" {
            w262 = string[] ["CameraPublisher", "Usage", "DB"]  # Items to initially close
            n137 = First Call?() -> (First Call?: T/F=w263:bool)
            n138 = control-ref of="Tree"() -> (w264:refnum<vi>)
            n139 = Select(t=w262, s=w263, f=string[] []) -> (s? t:f=w260:string[])
            n140 = call <vilib>:"NT Read and Format Entries as Tree.vi"("Tags to  Close"=w260, "Tree Refnum"=w264) -> ()  [unwired: 8 in, 2 out]
          }
          frame "Commands" {
            w273 = u32 5789784 ("Color Box")
            w274 = T25 {"Row"=-1, "Column"=-2} ("Active Cell:Active Cell")
            w276 = T25 {"Row"=-2, "Column"=-2} ("Active Cell:Active Cell")
            n141 = Index Array(array=w277, index=w271) -> (element=w275:u32)
            n142 = Index Array(array=w272, index=w271) -> (element=w270:T24)
            n143 = Unbundle(w270) -> ("Operation"=w269:enum16{"Update", "Clear"})  [unwired: 1 out]
            n144 = local read "Command Selection"() -> (w268:i32)
            n145 = property on="Command Selection" class="MCListbox (strict)"("ActiveCell"=w276, "CellBG"=w275, "ActiveCell"=w274, "CellBG"=w273) -> ()  [unwired: 2 in, 2 out]
            n146 = call <vilib>:"WPI_DashboardUpdate RPC Info.vi"("Operation"=w269) -> ("update"=w267:bool, "commands"=w266:string[][])  [unwired: 9 in]
            n147 = property on="Command Selection" class="MCListbox (strict)"("ItemNames"=w266) -> ()  [unwired: 2 in, 2 out]
            n148 = property on="Command Params" class="Tbl (strict)"("Active Cell"=w276, "Cell BG Color"=w275, "Active Cell"=w274, "Cell BG Color"=w273) -> ()  [unwired: 2 in, 2 out]
            n149 = call <vilib>:"WPI_DashboardUpdate Command Params.vi"("Update"=w267, "NewVal"=w268, "Commands"=w266, "Param Tbl"=w265) -> ()  [unwired: 7 in, 1 out]
          }
        }
        n150 = call <vilib>:"Connextion Info.vi"() -> ("Connected"=→"NT Connection":bool)  [unwired: 10 in, 1 out]
      }
      event "Test Tree": Value Change {
        # "Show appropriate\ncontrols"
        n151 = event-data() -> ("CtlRef"=w282:refnum<vi>, "NewVal"=w280:string)  [unwired: 1 in]
        n152 = call <vilib>:"WPI_UtilitiesGetTreeIOName.vi"("NewVal"=w280, "TreeControl in"=w282) -> ("I/O Name"=w283:string)  [unwired: 9 in]
        n153 = case shown="\"Camera\"" w283 {
          selector: w283 -> [_ w290 _ w312 w321 _]
          tunnel: w280 -> [_ _ w309 w311 _ w328]
          tunnel: cluster{string[]}[] [{["640x480", "320x240", "160x120"]}, {["Auto", "Fixed indoor", "Fixed outdoor 1", "Fixed outdoor 2", "Fixed fluorescent 1", "Fixed fluorescent 2", "Hold current"]}, {["Auto", "Flicker-free 50 Hz", "Flicker-free 60 Hz", "Hold current"]}, {["None", "Prioritize frame rate", "Prioritize image quality"]}, {["Monochrome", "Color"]}] -> [_ _ _ _ _ w327]
          frame Default {
            w285 = FALSE ("Visible")
            w284 = FALSE ("Visible")
            n154 = property on="Motor" class="Clust (strict)"("Visible"=w284) -> ()  [unwired: 2 in, 2 out]
            n155 = property on="Test Ring" class="Ring (strict)"("Visible"=w284) -> ()  [unwired: 2 in, 2 out]
            n156 = property on="Rev/Fwd" class="Clust (strict)"("Visible"=w285) -> ()  [unwired: 2 in, 2 out]
            n157 = property on="On/Off" class="Bool (strict)"("Visible"=w285) -> ()  [unwired: 2 in, 2 out]
            n158 = property on="Test Slider" class="Slide (strict)"("Visible"=w285) -> ()  [unwired: 2 in, 2 out]
          }
          frame "Analog Out", "Motor", "PWM" {
            w291 = FALSE ("Visible")
            n159 = case shown="\"Analog Out\"" w290 {
              tunnel: [1.0 ("Value") -1.0 ("Value") 0.0 ("Value")] -> w289
              tunnel: [255.0 ("Value") 1.0 ("Value") 5.0 ("Value")] -> w288
              tunnel: [128.0 ("Value") 0.0 ("Value") 0.0 ("Value")] -> w287
              tunnel: [64.0 ("Value") 0.5 ("Value") 1.0 ("Value")] -> w286
              frame "PWM" {
              }
              frame "Motor", Default {
              }
              frame "Analog Out" {
              }
            }
            n160 = property on="Motor" class="Clust (strict)"("Visible"=TRUE) -> ()  [unwired: 2 in, 2 out]
            n161 = property on="Value" class="Slide (strict)"("Value"=w287, "Scale.Minimum"=w289, "Scale.Maximum"=w288, "Scale.Increment"=w286) -> ()  [unwired: 2 in, 2 out]
            n162 = property on="On/Off" class="Bool (strict)"("Visible"=w291) -> ()  [unwired: 2 in, 2 out]
            n163 = property on="Test Slider" class="Slide (strict)"("Visible"=w291) -> ()  [unwired: 2 in, 2 out]
            n164 = property on="Test Ring" class="Ring (strict)"("Visible"=w291) -> ()  [unwired: 2 in, 2 out]
            n165 = property on="Rev/Fwd" class="Clust (strict)"("Visible"=w291) -> ()  [unwired: 2 in, 2 out]
          }
          frame "Servo" {
            w307 = FALSE ("Visible")
            n166 = call <vilib>:"NT Read Number.vi"("Name"=w309) -> ("Numeric"=w308:dbl)  [unwired: 9 in, 1 out]
            n167 = property on="Test Slider" class="Slide (strict)"("Visible"=TRUE, "Scale.Maximum"=170.0 ("Scale.Range:Maximum")) -> ()  [unwired: 2 in, 2 out]
            n168 = local write "Test Slider"(w308) -> ()
            n169 = property on="Motor" class="Clust (strict)"("Visible"=w307) -> ()  [unwired: 2 in, 2 out]
            n170 = property on="Rev/Fwd" class="Clust (strict)"("Visible"=w307) -> ()  [unwired: 2 in, 2 out]
            n171 = property on="On/Off" class="Bool (strict)"("Visible"=w307) -> ()  [unwired: 2 in, 2 out]
            n172 = property on="Test Ring" class="Ring (strict)"("Visible"=w307) -> ()  [unwired: 2 in, 2 out]
          }
          frame "Relay", "Solenoid" {
            w310 = FALSE ("Visible")
            n173 = property on="Motor" class="Clust (strict)"("Visible"=w310) -> ()  [unwired: 2 in, 2 out]
            n174 = property on="Test Slider" class="Slide (strict)"("Visible"=w310) -> ()  [unwired: 2 in, 2 out]
            n175 = Search and Replace String(input string=w311, search string="/Value  **", replace string="/Direction") -> (result string=w317:string)  [unwired: 5 in, 3 out]
            n176 = property on="Test Ring" class="Ring (strict)"("Visible"=w310) -> ()  [unwired: 2 in, 2 out]
            n177 = call <vilib>:"NT Read String.vi"("Name"=w317) -> ("String"=w315:string)  [unwired: 9 in, 1 out]
            n178 = Equal?(x="Both directions", y=w315) -> (x = y?=w313:bool)
            n179 = Not(x=w313) -> (.not. x?=w314:bool)
            n180 = property on="Rev/Fwd" class="Clust (strict)"("Visible"=w313) -> ()  [unwired: 2 in, 2 out]
            n181 = property on="On/Off" class="Bool (strict)"("Visible"=w314, "Caption.Text"=w312) -> ()  [unwired: 2 in, 2 out]
          }
          frame "Compressor", "Digital Out" {
            w320 = FALSE ("Visible")
            # "Get direction and finish"
            n182 = property on="Motor" class="Clust (strict)"("Visible"=w320) -> ()  [unwired: 2 in, 2 out]
            n183 = property on="Test Slider" class="Slide (strict)"("Visible"=w320) -> ()  [unwired: 2 in, 2 out]
            n184 = property on="Test Ring" class="Ring (strict)"("Visible"=w320) -> ()  [unwired: 2 in, 2 out]
            n185 = property on="On/Off" class="Bool (strict)"("Visible"=TRUE, "Caption.Text"=w321) -> ()  [unwired: 2 in, 2 out]
            n186 = property on="Rev/Fwd" class="Clust (strict)"("Visible"=FALSE) -> ()  [unwired: 2 in, 2 out]
          }
          frame "Camera" {
            n187 = call <vilib>:"Get Last Path Segment.vi"("String in"=w328) -> ("String out"=w329:string)  [unwired: 10 in]
            n188 = property on="On/Off" class="Bool (strict)"("Visible"=FALSE) -> ()  [unwired: 2 in, 2 out]
            n189 = property on="Motor" class="Clust (strict)"("Visible"=FALSE) -> ()  [unwired: 2 in, 2 out]
            n190 = property on="Rev/Fwd" class="Clust (strict)"("Visible"=FALSE) -> ()  [unwired: 2 in, 2 out]
            n191 = case shown="\"White Balance  **\"" w329 {
              tunnel: w328 -> [w335 w344 w353 w362 w371 _ w377]
              tunnel: w327 -> [w333 w341 w350 w359 w368 _ _]
              frame "Size  **" {
                n192 = Index Array(array=w333) -> (element=w332:cluster{string[]})  [unwired: 1 in]
                n193 = call <vilib>:"NT Read String.vi"("Name"=w335) -> ("String"=w334:string)  [unwired: 9 in, 1 out]
                n194 = Unbundle(w332) -> (w330:string[])
                n195 = Match First String(2:w330, 3:w334) -> (0:w331:i32)  [unwired: 1 out]
                n196 = property on="Test Ring" class="Ring (strict)"("Value"=w331, "Strings []"=w330) -> ()  [unwired: 2 in, 2 out]
                n197 = property on="Test Ring" class="Ring (strict)"("Visible"=TRUE) -> ()  [unwired: 2 in, 2 out]
                n198 = property on="Test Slider" class="Slide (strict)"("Visible"=FALSE) -> ()  [unwired: 2 in, 2 out]
              }
              frame "White Balance  **" {
                n199 = Index Array(array=w341, index=1) -> (element=w342:cluster{string[]})
                n200 = call <vilib>:"NT Read String.vi"("Name"=w344) -> ("String"=w343:string)  [unwired: 9 in, 1 out]
                n201 = Unbundle(w342) -> (w339:string[])
                n202 = Match First String(2:w339, 3:w343) -> (0:w338:i32)  [unwired: 1 out]
                n203 = property on="Test Ring" class="Ring (strict)"("Value"=w338, "Strings []"=w339) -> ()  [unwired: 2 in, 2 out]
                n204 = property on="Test Ring" class="Ring (strict)"("Visible"=TRUE) -> ()  [unwired: 2 in, 2 out]
                n205 = property on="Test Slider" class="Slide (strict)"("Visible"=FALSE) -> ()  [unwired: 2 in, 2 out]
              }
              frame "Exposure  **" {
                n206 = Index Array(array=w350, index=2) -> (element=w351:cluster{string[]})
                n207 = call <vilib>:"NT Read String.vi"("Name"=w353) -> ("String"=w352:string)  [unwired: 9 in, 1 out]
                n208 = Unbundle(w351) -> (w347:string[])
                n209 = Match First String(2:w347, 3:w352) -> (0:w348:i32)  [unwired: 1 out]
                n210 = property on="Test Ring" class="Ring (strict)"("Value"=w348, "Strings []"=w347) -> ()  [unwired: 2 in, 2 out]
                n211 = property on="Test Ring" class="Ring (strict)"("Visible"=TRUE) -> ()  [unwired: 2 in, 2 out]
                n212 = property on="Test Slider" class="Slide (strict)"("Visible"=FALSE) -> ()  [unwired: 2 in, 2 out]
              }
              frame "Exposure Priority  **" {
                n213 = Index Array(array=w359, index=3) -> (element=w360:cluster{string[]})
                n214 = call <vilib>:"NT Read String.vi"("Name"=w362) -> ("String"=w361:string)  [unwired: 9 in, 1 out]
                n215 = Unbundle(w360) -> (w356:string[])
                n216 = Match First String(2:w356, 3:w361) -> (0:w357:i32)  [unwired: 1 out]
                n217 = property on="Test Ring" class="Ring (strict)"("Value"=w357, "Strings []"=w356) -> ()  [unwired: 2 in, 2 out]
                n218 = property on="Test Ring" class="Ring (strict)"("Visible"=TRUE) -> ()  [unwired: 2 in, 2 out]
                n219 = property on="Test Slider" class="Slide (strict)"("Visible"=FALSE) -> ()  [unwired: 2 in, 2 out]
              }
              frame "Color Enable  **" {
                n220 = Index Array(array=w368, index=4) -> (element=w369:cluster{string[]})
                n221 = call <vilib>:"NT Read String.vi"("Name"=w371) -> ("String"=w370:string)  [unwired: 9 in, 1 out]
                n222 = Unbundle(w369) -> (w365:string[])
                n223 = Match First String(2:w365, 3:w370) -> (0:w366:i32)  [unwired: 1 out]
                n224 = property on="Test Ring" class="Ring (strict)"("Value"=w366, "Strings []"=w365) -> ()  [unwired: 2 in, 2 out]
                n225 = property on="Test Ring" class="Ring (strict)"("Visible"=TRUE) -> ()  [unwired: 2 in, 2 out]
                n226 = property on="Test Slider" class="Slide (strict)"("Visible"=FALSE) -> ()  [unwired: 2 in, 2 out]
              }
              frame Default {
                n227 = property on="Test Ring" class="Ring (strict)"("Visible"=FALSE) -> ()  [unwired: 2 in, 2 out]
                n228 = property on="Test Slider" class="Slide (strict)"("Visible"=FALSE) -> ()  [unwired: 2 in, 2 out]
              }
              frame "Brightness  **", "Color Level  **", "Compression  **", "FPS  **", "Sharpness  **" {
                n229 = call <vilib>:"NT Read Number.vi"("Name"=w377) -> ("Numeric"=w376:dbl)  [unwired: 9 in, 1 out]
                n230 = local write "Test Slider"(w376) -> ()
                n231 = property on="Test Slider" class="Slide (strict)"("Visible"=TRUE, "Scale.Maximum"=100.0 ("Scale.Range:Maximum")) -> ()  [unwired: 2 in, 2 out]
                n232 = property on="Test Ring" class="Ring (strict)"("Visible"=FALSE) -> ()  [unwired: 2 in, 2 out]
              }
            }
          }
        }
        n233 = property on="Progress" class="Clust (strict)"("Visible"=FALSE) -> ()  [unwired: 2 in, 2 out]
      }
      event "Test Name": Mouse Enter {
        # "Populate the ring with the list of tests"
        n234 = event-data() -> ()  [unwired: 1 in, 1 out]
        n235 = call <vilib>:"NT Read String Array.vi"("Name"="TestMode/TestList") -> ("String Array"=w385:string[])  [unwired: 9 in, 1 out]
        n236 = Build Array (concatenate)("Select the test to run...", w385) -> (w384:string[])
        n237 = property on="Test Name" class="Ring (strict)"("Strings []"=w384) -> ()  [unwired: 2 in, 2 out]
      }
      event "Test Name": Value Change {
        w387 = FALSE ("Visible")
        # "Tell the robot the test name to run"
        n238 = event-data() -> ("NewVal"=w391:u16)  [unwired: 1 in]
        n239 = property on="Test Name" class="Ring (strict)"() -> ("Strings []"=w392:string[])  [unwired: 2 in, 2 out]
        n240 = local write "Progress"(T6 {"Test Progress"=0, "Test Progress Text"=""} ("Progress")) -> ()
        n241 = Index Array(array=w392, index=w391) -> (element=w390:string)
        n242 = call <vilib>:"NT Write String.vi"("String"=w390, "Name"="TestMode/TestName") -> ()  [unwired: 9 in, 1 out]
        n243 = property on="Progress" class="Clust (strict)"("Visible"=TRUE) -> ()  [unwired: 2 in, 2 out]
        n244 = property on="Motor" class="Clust (strict)"("Visible"=w387) -> ()  [unwired: 2 in, 2 out]
        n245 = property on="Test Slider" class="Slide (strict)"("Visible"=w387) -> ()  [unwired: 2 in, 2 out]
        n246 = property on="On/Off" class="Bool (strict)"("Visible"=w387) -> ()  [unwired: 2 in, 2 out]
        n247 = property on="Rev/Fwd" class="Clust (strict)"("Visible"=w387) -> ()  [unwired: 2 in, 2 out]
        n248 = property on="Test Ring" class="Ring (strict)"("Visible"=w387) -> ()  [unwired: 2 in, 2 out]
      }
      event "Select Auto": Mouse Enter {
        # "Populate the combo box with the list of autonomous options"
        n249 = event-data() -> ()  [unwired: 1 in, 1 out]
        n250 = call <vilib>:"NT Read String Array.vi"("Name"="Auto List") -> ("String Array"=w394:string[])  [unwired: 9 in, 1 out]
        n251 = property on="Select Auto" class="CmbBox"("Strings[]"=w394) -> ()  [unwired: 2 in, 2 out]
      }
      event "Select Auto": Value Change {
        # "User modified the Auto Selection. Write to NT variable so robot knows."
        n252 = event-data() -> ("NewVal"=w397:string)  [unwired: 1 in]
        n253 = call <vilib>:"NT Write String.vi"("String"=w397, "Name"="Auto Selector") -> ()  [unwired: 9 in, 1 out]
      }
      event "Command Selection": Value Change {
        # "Get the params and show in table"
        n254 = event-data() -> ("NewVal"=w403:i32)  [unwired: 1 in]
        n255 = property on="Command Selection" class="MCListbox (strict)"() -> ("ItemNames"=w401:string[][])  [unwired: 2 in, 2 out]
        n256 = call <vilib>:"WPI_DashboardUpdate Command Params.vi"("NewVal"=w403, "Commands"=w401, "Param Tbl"=w402) -> ()  [unwired: 8 in, 1 out]
      }
      event "Execute Command": Value Change {
        # "Started one, Unique ID holds\nresponse"
        n257 = event-data() -> ()  [unwired: 1 in, 1 out]
        n258 = property on="Command Selection" class="MCListbox (strict)"() -> ("ItemNames"=w414:string[][])  [unwired: 2 in, 2 out]
        n259 = Index Array(array=w414, index (row)="Command Selection", index (col)=0) -> (element=w412:string)
        n260 = call <vilib>:"Invoke Commands.vi"("Command Params"="Command Params", "Function Name"=w412) -> ("Params"=w408:u8, "Started"=w407:bool)  [unwired: 7 in, 1 out]
        n261 = Array Subset(array="Command Params", length (row)=w408) -> (w409:string[][])  [unwired: 3 in]
        n262 = Select(t="Executing" ("Cmd Status"), s=w407, f="" ("Cmd Status")) -> (s? t:f=→"Cmd Status":string)
      }
      event "Command Selection": Double Click {
        n263 = event-data() -> ("Row"=w422:i32)  [unwired: 1 in]
        n264 = property on="Command Selection" class="MCListbox (strict)"() -> ("ItemNames"=w425:string[][])  [unwired: 2 in, 2 out]
        n265 = local read "Command Params"() -> (w421:string[][])
        n266 = Index Array(array=w425, index (row)=w422, index (col)=0) -> (element=w423:string)
        n267 = call <vilib>:"Invoke Commands.vi"("Command Params"=w421, "Function Name"=w423) -> ("Params"=w420:u8, "Started"=w415:bool)  [unwired: 7 in, 1 out]
        n268 = Array Subset(array=w421, length (row)=w420) -> (w419:string[][])  [unwired: 3 in]
        n269 = Select(t="Executing" ("Cmd Status"), s=w415, f="" ("Cmd Status")) -> (s? t:f=w416:string)
        n270 = local write "Cmd Status"(w416) -> ()
      }
      event "CheckList": Double Click {
        # "Shift clears all"
        # "Update symbols on the listbox"
        n271 = event-data() -> ("PlatMods.Shift"=w427:bool, "Row"=w429:i32)  [unwired: 1 in]
        n272 = case shown="True" w427 {
          tunnel: w429 -> [w433 _]
          tunnel: 1 -> [w432 _]
          frame False {
            n273 = property on="CheckList" class="LstBox (strict)"() -> ("Item Symbols"=w431:i32[])  [unwired: 2 in, 2 out]
            n274 = Replace Array Subset(array=w431, new element=w432, index=w433) -> (w430:i32[])
            n275 = property on="CheckList" class="LstBox (strict)"("Item Symbols"=w430) -> ()  [unwired: 2 in, 2 out]
          }
          frame True {
            w434 = 0 ("Top Row")
            n276 = property on="CheckList" class="LstBox (strict)"() -> ("Number of Rows"=w436:u32)  [unwired: 2 in, 2 out]
            n277 = Initialize Array(0, w436) -> (w435:i32[])
            n278 = property on="CheckList" class="LstBox (strict)"("Top Row"=w434, "Value"=w434, "Item Symbols"=w435) -> ()  [unwired: 2 in, 2 out]
          }
        }
      }
      event "CheckList": Key Down {
        # "Update symbols on the listbox\nLeft and right keys check and uncheck"
        n279 = event-data() -> ("VKey"=w440:T22)  [unwired: 1 in]
        n280 = case shown="\"Left\", \"Right\"" w440 {
          selector: w440 -> [w445 _]
          tunnel: eventvkey."Left" ("VKey") -> [w443 _]
          frame "Left", "Right" {
            n281 = Equal?(x=w443, y=w445) -> (x = y?=w444:bool)
            n282 = Select(t=0, s=w444, f=1) -> (s? t:f=w446:i32)
            n283 = property on="CheckList" class="LstBox (strict)"() -> ("Item Symbols"=w449:i32[])  [unwired: 2 in, 2 out]
            n284 = Replace Array Subset(array=w449, new element=w446, index="CheckList") -> (w448:i32[])
            n285 = property on="CheckList" class="LstBox (strict)"("Item Symbols"=w448) -> ()  [unwired: 2 in, 2 out]
          }
          frame Default {
          }
        }
      }
      event "Motor.Enable": Value Change {
        # "When the test mode otor enable helper is set, update that\ntree row item's value"
        n286 = event-data() -> ("NewVal"=w455:bool)  [unwired: 1 in]
        n287 = Unbundle("Motor") -> ("Value"=w454:dbl)  [unwired: 1 out]
        n288 = Select(t=w454, s=w455, f=0.0) -> (s? t:f=w452:dbl)
        n289 = call <vilib>:"NT Write Number.vi"("Numeric"=w452, "Name"=w451) -> ()  [unwired: 9 in, 1 out]
      }
      event "Test Slider": Value Change {
        # "When the test mode slider helper is set, update that\ntree row item's value"
        n290 = event-data() -> ("NewVal"=w458:dbl)  [unwired: 1 in]
        n291 = call <vilib>:"NT Write Number.vi"("Numeric"=w458, "Name"=w459) -> ()  [unwired: 9 in, 1 out]
      }
      event "On/Off": Value Change {
        # "When the test mode on/off helper value is set, update that\ntree row item's value"
        n292 = event-data() -> ("NewVal"=w463:bool)  [unwired: 1 in]
        n293 = Boolean To (0,1)(Boolean=w463) -> (0, 1=w462:i16)
        n294 = call <vilib>:"NT Write Number.vi"("Numeric"=w462, "Name"=w461) -> ()  [unwired: 9 in, 1 out]
      }
      event "Rev/Fwd": Value Change {
        # "When the test mode helper value for relays is set, update that\ntree row item's value"
        n295 = event-data() -> ("NewVal.Forward"=w471:bool, "NewVal.Reverse"=w470:bool)  [unwired: 1 in]
        n296 = Boolean To (0,1)(Boolean=w471) -> (0, 1=w467:i16)
        n297 = Boolean To (0,1)(Boolean=w470) -> (0, 1=w469:i16)
        n298 = Negate(x=w469) -> (-x=w468:i16)
        n299 = Add(x=w467, y=w468) -> (x+y=w466:i16)
        n300 = call <vilib>:"NT Write Number.vi"("Numeric"=w466, "Name"=w465) -> ()  [unwired: 9 in, 1 out]
      }
      event "Test Ring": Value Change {
        # "When a test mode helper value is selected from the ring,\nset the tree item's variable to the string value"
        n301 = event-data() -> ("NewVal"=w475:u16)  [unwired: 1 in]
        n302 = property on="Test Ring" class="Ring (strict)"() -> ("Strings []"=w476:string[])  [unwired: 2 in, 2 out]
        n303 = Index Array(array=w476, index=w475) -> (element=w474:string)
        n304 = call <vilib>:"NT Write String.vi"("String"=w474, "Name"=w473) -> ()  [unwired: 9 in, 1 out]
      }
      event "Rec Mode": Value Change {
        # "Update globals for recording mode and path to read log from.\nClear when logging and let NetworkTables set path for vision to\nuse."
        n305 = event-data() -> ("NewVal"=w487:enum32{"Stop", "Record", "Playback"})  [unwired: 1 in]
        n306 = global write "WPI_DashboardLogging Global.vi" "Logging Filename"(path "") -> ()
        n307 = global write "WPI_DashboardLogging Global.vi" "Recording"(w487) -> ()
        n308 = case shown="\"Playback\"" w487 {
          tunnel: w486 -> [_ w489 w498]
          tunnel: [_ _ w497] -> w484
          tunnel: [_ _ w496] -> _
          tunnel: w482 -> [_ _ w494]
          tunnel: cluster{i32, i32} {-250, 170} -> [_ _ w493]
          tunnel: [_ _ T23 {"Image Size"=TRUE, "Image Type"=TRUE, "Pixel Value"=TRUE, "ROI Information"=TRUE, "Zoom Factor"=FALSE} ("Image Information Shown:All Elements")] -> w477
          tunnel: [_ _ TRUE ("Zoom Factor")] -> w478
          tunnel: w480 -> [_ _ w490]
          frame Default {
          }
          frame "Stop", "Record" {
            # "Place Window too"
            n309 = invoke class="VI" method="FP.Close"(reference=w489) -> (reference out=w488:refnum<vi>)  [unwired: 2 in, 2 out]
            n310 = invoke class="VI" method="Abort VI"(reference=w488) -> ()  [unwired: 2 in, 3 out]
          }
          frame "Playback" {
            n311 = call "Open Playback Panel.vi"("Offset"=w493, "DB VI Ref"=w494, "Playback in"=w498) -> ("Playback out"=w495:refnum<vi>)  [unwired: 8 in]
            n312 = register-events(w495, w490) -> (reference out=w497:refnum<event-registration>, error out=w496:errorcluster)  [unwired: 2 in]
          }
        }
        n313 = property on="Camera Image Right" class="ImageControl"("Image Information Shown"=w477, "Image Information Visible"=w478) -> ()  [unwired: 2 in, 2 out]
        n314 = property on="Camera Image" class="ImageControl"("Image Information Shown"=w477, "Image Information Visible"=w478) -> ()  [unwired: 2 in, 2 out]
        n315 = call <vilib>:"WPI_DashboardNT Log FieldName Cache.vi"("Operation"=enum16{"Lookup/Add", "Index", "Clear"}."Clear") -> ()  [unwired: 8 in, 3 out]
      }
      event Panel Close {
        w500 = enum32{"Stop", "Record", "Playback"}."Stop" ("Rec Mode")
        # "Playback window has been closed, abort"
        n316 = event-data() -> ()  [unwired: 1 in, 4 out]
        n317 = local write "Rec Mode"(w500) -> ()
        n318 = global write "WPI_DashboardLogging Global.vi" "Recording"(w500) -> ()
      }
      event Panel Close {
        # "Abort playback window and ourself"
        n319 = event-data() -> ()  [unwired: 1 in, 4 out]
        n320 = invoke class="VI" method="FP.Close"(reference=w504) -> (reference out=w503:refnum<vi>)  [unwired: 2 in, 2 out]
        n321 = invoke class="VI" method="Abort VI"(reference=w503) -> (error out=w502:errorcluster)  [unwired: 2 in, 2 out]
        n322 = invoke class="VI" method="Abort VI"(error in=w502) -> ()  [unwired: 2 in, 3 out]
      }
      event User Event {
        n323 = event-data() -> ("IDs"=w511:cluster{"RPC field ID":u16, "Unique ID":u16}, "String"=w510:string)  [unwired: 1 in]
        n324 = Bundle("IDs"=w511, "String"=w510) -> (w509:T10)  [unwired: 1 in]
        n325 = call <vilib>:"Retrieve RPC Response.vi"("RPC Response"=w509) -> ("Output"=w507:string[][])  [unwired: 10 in]
        n326 = Build Array (concatenate)(w505, w507) -> (w506:string[][])
        n327 = local write "Command Params"(w506) -> ()
        n328 = local write "Cmd Status"("" ("Cmd Status")) -> ()
      }
      event "Tree": Double Click {
        n329 = event-data() -> ("PlatMods"=w517:T26, "Tag"=w514:string)  [unwired: 1 in]
        n330 = Unbundle(w517) -> ("Shift"=w516:bool)  [unwired: 4 out]
        n331 = String Subset(string=w514, length (rest)=1 ("length (rest)")) -> (substring=w513:string)  [unwired: 1 in]
        n332 = Not(x=w516) -> (.not. x?=w515:bool)
        n333 = case shown="\"/\"" w513 {
          tunnel: w514 -> [_ w520]
          tunnel: w515 -> [_ w519]
          frame Default {
          }
          frame "/" {
            n334 = call <vilib>:"NT Update Persistence.vi"("Persistence"=w519, "Name"=w520) -> ()  [unwired: 9 in, 1 out]
          }
        }
      }
    }
  }
  n335 = while {
    tunnel: w63 -> [w522]
    i -> [w525]
    stop <- FALSE stop-if-true
    n336 = Wait (ms)(milliseconds to wait=u32 100) -> ()  [unwired: 1 out]
    n337 = case shown="\"Stop\", Default" "Rec Mode" {
      tunnel: w525 -> [_ _ w540]
      tunnel: [u32 2829099 ("Base Color") u32 11141120 ("Target Color") w529] -> w521
      frame "Stop", Default {
        # "Reset the color, extra updates don't cost much"
      }
      frame "Record" {
      }
      frame "Playback" {
        # "Playback"
        n338 = Quotient & Remainder(x=w540, y=u32 50 ("milliseconds to wait")) -> (x-y*floor(x/y)=w536:u32)  [unwired: 1 out]
        n339 = Divide(x=w536, y=u32 50 ("milliseconds to wait")) -> (x/y=w533:dbl)
        n340 = Multiply(x=6.283185307179586, y=w533) -> (x*y=w538:dbl)
        n341 = Sine(x=w538) -> (sin(x)=w537:dbl)
        n342 = Absolute Value(x=w537) -> (abs(x)=w530:dbl)
        n343 = call "Interpolate RGB Color.vi"("Proportion"=w530, "Target Color"=u32 30976, "Base Color"=u32 2829099) -> ("Result Color"=w529:u32)  [unwired: 8 in]
      }
    }
    n344 = property class="Pane"(reference=w522, "PaneColor"=w521) -> ()  [unwired: 1 in, 2 out]
  }
  n345 = local write "Dashboard Tab"(T2."Drive" ("Dashboard Tab")) -> ()
  n346 = property on="On/Off" class="Bool (strict)"("Visible"=w40) -> ()  [unwired: 2 in, 2 out]
  n347 = property on="Motor" class="Clust (strict)"("Visible"=w40) -> ()  [unwired: 2 in, 2 out]
  n348 = property on="Progress" class="Clust (strict)"("Visible"=w40) -> ()  [unwired: 2 in, 2 out]
  n349 = property on="Test Ring" class="Ring (strict)"("Visible"=w40) -> ()  [unwired: 2 in, 2 out]
  n350 = property on="Rev/Fwd" class="Clust (strict)"("Visible"=w40) -> ()  [unwired: 2 in, 2 out]
  n351 = local write "Command Selection"(u16 0 ("milliseconds to wait")) -> ()
  n352 = local write "Command Params"(string[][] [] ("Command Params")) -> ()
  n353 = while {
    tunnel: u16 1741 ("timeout ms (25000)") -> [w542]
    stop <- FALSE stop-if-true
    n354 = TCP Create Listener(10:w542) -> (0:w541:errorcluster, 3:w543:refnum<k5>)  [unwired: 4 in, 1 out]
    n355 = case shown="Error" w541 {
      selector: w541 -> [w545 _]
      tunnel: w543 -> [w546 _]
      frame No Error {
        n356 = while {
          tunnel: w546 -> [w549]
          tunnel: w545 -> [w548]
          stop <- FALSE stop-if-true
          n357 = TCP Wait On Listener(8:w548, 11:w549) -> (0:w550:errorcluster, 4:w551:refnum<k5>)  [unwired: 2 in, 3 out]
          n358 = local write "TCP"(w551) -> ()
          n359 = case shown="No Error" w550 {
            frame No Error {
            }
            frame Error {
              n360 = Wait (ms)(milliseconds to wait=u32 1000) -> ()  [unwired: 1 out]
            }
          }
        }
      }
      frame Error {
        n361 = Wait (ms)(milliseconds to wait=u32 1000) -> ()  [unwired: 1 out]
      }
    }
  }
  n362 = global write "WPI_DashboardLogging Global.vi" "Recording"(w57) -> ()
  n363 = local write "Rec Mode"(w57) -> ()
  n364 = call <vilib>:"NT Write String.vi"("String"="Select Auto", "Name"="Auto Selector") -> ()  [unwired: 9 in, 1 out]
